vi "Write Bus Busy Time (us).vi"(8 "error in (no error)":errorcluster, 10 "Bus Busy Time (us)":u64, 11 "GenBus_Load_Calculator in":refnum<class "GenBus_Load_Calculator.lvclass">) -> (0 "error out":errorcluster, 3 "GenBus_Load_Calculator out":refnum<class "GenBus_Load_Calculator.lvclass">)   [LabVIEW 2019, in "XNET-Bus-Load-Calculator.lvlib" / "GenBus_Load_Calculator.lvclass"]
uses:
  GenBus_Load_Calculator.lvclass
  GenBus_Load_Calculator.lvclass/GenBus_Load_Calculator.ctl
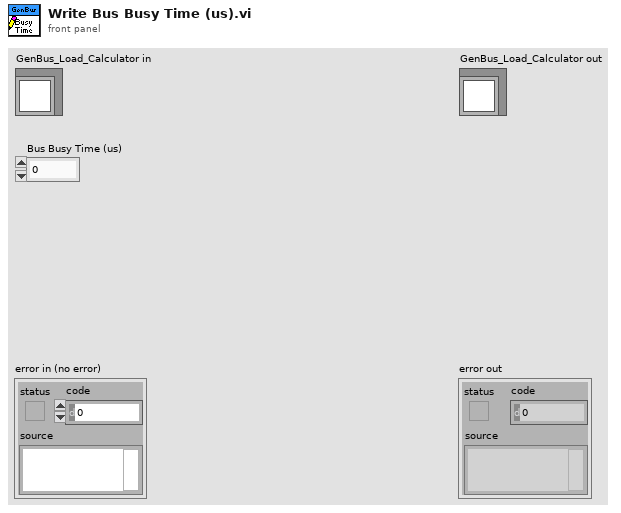
[diagram p1: front panel]
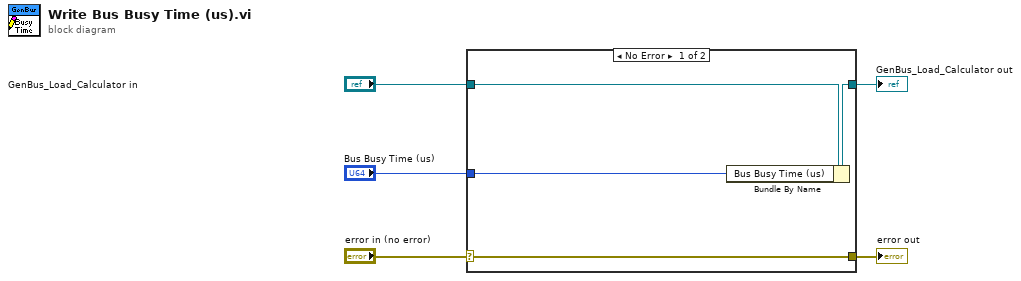
[diagram p0: block diagram]
diagram:
  n1 = case shown="No Error" "error in (no error)" {
    selector: "error in (no error)" -> [w9 w10]
    tunnel: [w9 w10] -> w4
    tunnel: [w7 w11] -> w2
    tunnel: "GenBus_Load_Calculator in" -> [w8 w11]
    tunnel: "Bus Busy Time (us)" -> [w6 _]
    frame No Error {
      n2 = Bundle By Name(cluster=w8, "Bus Busy Time (us)"=w6) -> (w7:refnum<class "GenBus_Load_Calculator.lvclass">)
    }
    frame Error {
    }
  }
  "error out" <- w4
  "GenBus_Load_Calculator out" <- w2
